vi "Update_DAQmxTask_value.vi"(8 "error in (no error)":errorcluster, 9 "Value":bool, 10 "Task name":string, 11 "DAQmxTaksContainer_General in":refnum<class "DAQmxTaksContainer_General.lvclass">) -> (0 "error out":errorcluster, 3 "DAQmxTaksContainer_General out":refnum<class "DAQmxTaksContainer_General.lvclass">)   [LabVIEW 2019, in "DAQmxTaksContainer_General.lvclass"]
uses:
  DAQmxTaksContainer_General.lvclass
  DAQmxTaksContainer_General.lvclass/DAQmxTaksContainer_General.ctl
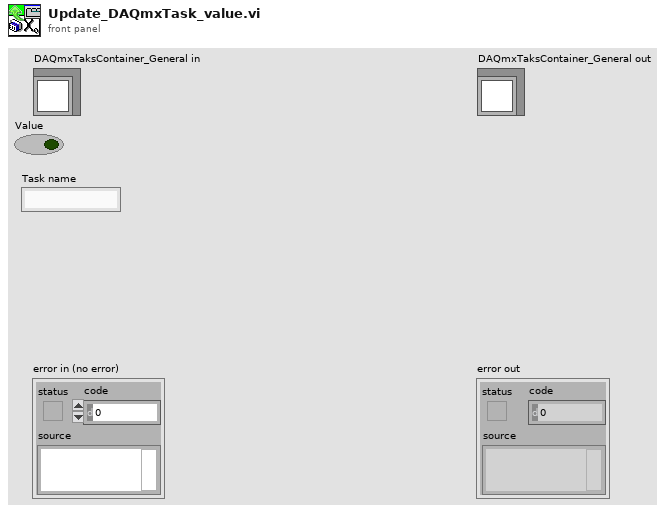
[diagram p1: front panel]
types:
  T1 = cluster{"name":string, "type of task":string, "Status":bool, "Value":string, "error":errorcluster}[]
  T2 = cluster{"name":string, "type of task":string, "Status":bool, "Value":string, "error":errorcluster}
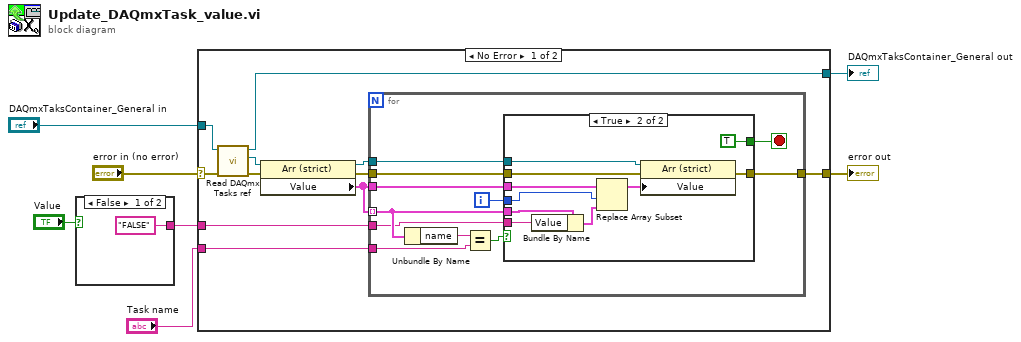
[diagram p0: block diagram]
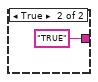
[diagram p2: hidden frame]
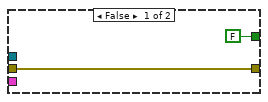
[diagram p3: hidden frame]
diagram:
  n1 = case shown="False" "Value" {
    tunnel: ["FALSE" "TRUE"] -> w1
    frame False {
    }
    frame True {
    }
  }
  n2 = case shown="No Error" "error in (no error)" {
    selector: "error in (no error)" -> [w13 w45]
    tunnel: [w11 w45] -> w6
    tunnel: [w15 w44] -> w4
    tunnel: "DAQmxTaksContainer_General in" -> [w16 w44]
    tunnel: "Task name" -> [w14 _]
    tunnel: w1 -> [w10 _]
    frame No Error {
      n3 = call "Read DAQmx Tasks ref.vi"("error in (no error)"=w13, "DAQmxTaksContainer_General in"=w16) -> ("error out"=w19:errorcluster, "DAQmx Tasks ref"=w20:refnum<vi>, "DAQmxTaksContainer_General out"=w15:refnum<class "DAQmxTaksContainer_General.lvclass">)  [unwired: 7 in]
      n4 = property class="Arr (strict)"(reference=w20, error in=w19) -> (reference out=w18:refnum<vi>, error out=w12:errorcluster, "Value"=w17:T1)
      n5 = for {
        tunnel: w17 -> [w28] mode=indexing
        tunnel: w14 -> [w31]
        tunnel: w10 -> [w27]
        tunnel: w17 -> [w25]
        tunnel: w18 -> [w24]
        tunnel: w12 -> [w22]
        tunnel: [w21] -> w11
        i -> [w23]
        stop <- w26 stop-if-true
        n6 = Unbundle By Name(w28) -> ("name"=w29:string)
        n7 = Equal?(x=w29, y=w31) -> (x = y?=w30:bool)
        n8 = case shown="True" w30 {
          tunnel: w28 -> [_ w43]
          tunnel: w27 -> [_ w42]
          tunnel: [FALSE TRUE] -> w26
          tunnel: w25 -> [_ w38]
          tunnel: w24 -> [_ w37]
          tunnel: w23 -> [_ w36]
          tunnel: w22 -> [w32 w35]
          tunnel: [w32 w34] -> w21
          frame False {
          }
          frame True {
            n9 = Bundle By Name(cluster=w43, "Value"=w42) -> (w41:T2)
            n10 = Replace Array Subset(array=w38, new element=w41, index=w36) -> (w39:T1)
            n11 = property class="Arr (strict)"(reference=w37, error in=w35, "Value"=w39) -> (error out=w34:errorcluster)  [unwired: 1 out]
          }
        }
      }
    }
    frame Error {
    }
  }
  "error out" <- w6
  "DAQmxTaksContainer_General out" <- w4
